vi "Process.vi"(8 "error in":errorcluster, 11 "DAQmx-AI":refnum<class "DAQmx-AI.lvclass">) -> (0 "error out":errorcluster, 3 "DAQmx-AI out":refnum<class "DAQmx-AI.lvclass">)   [LabVIEW 2016, in "DAQmx-AI.lvclass"]
doc: "---------------------------------------------------------------\nJKI State Machine Objects™\nhttp://jki.net/state-machine-objects/\nCopyright (C) 2005-2015, JKI <info@jki.net>\nALL RIGHTS RESERVEDJKI State Machine Objects (SMO) 1.0.0.5\nJKI - JKI\nCopyright (c) 2016, JKI"
uses:
  DAQmx-AI.lvclass
  C:/Program Files (x86)/National Instruments/LabVIEW 2016/vi.lib/JKI/JKI SMO/SMO/SMO.lvclass
  <vilib>/JKI/JKI SMO/SMO/Typedefs/Parent Call--Enum.ctl
  <vilib>/Platform/TimedLoop/XDataNode/timing_clust.ctl
  <vilib>/Platform/TimedLoop/XDataNode/nitl_modes.ctl
  <vilib>/Platform/TimedLoop/XDataNode/wakeup.ctl
  <vilib>/DAQmx/read.llb/DAQmx Read (Analog Wfm 1Chan NSamp).vi
  <vilib>/DAQmx/miscellaneous.llb/DAQmx Fill In Error Info.vi
  <vilib>/platform/TimedLoop/XDataNode/XDataNode.xnode
  <vilib>/JKI/JKI SMO/SMO/SMO.lvclass
  <vilib>/Platform/TimedLoop/XDataNode/XDNodeRunTimeDep.lvlib
panel:
  out "Chart":waveform(dbl)(graph)
  # "For instructions on how to use the JKI State Machine Objects, examples and video tutorials, visit:\nhttp://jki.net/state-machine-objects/\n\nJKI State Machine Objects™\nhttp://jki.net/state-machine-objects/\nCopyright (C) 2005-2015, JKI <info@jki.net>\nALL RIGHTS RESERVED"
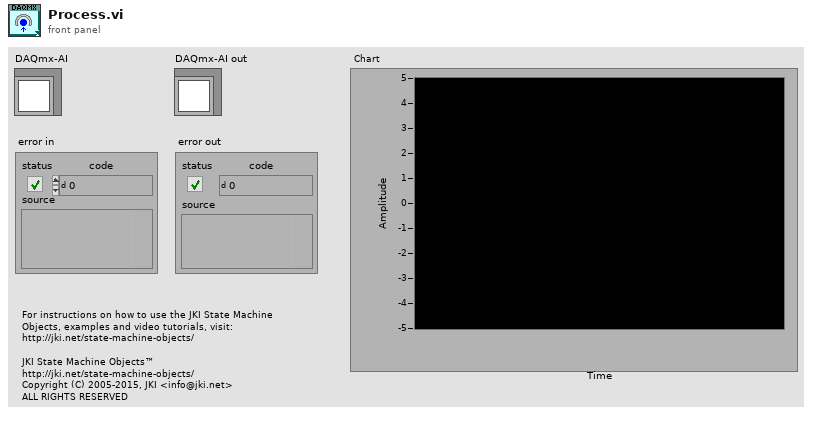
[diagram p1: front panel]
types:
  T1 = typedef "SMO.lvclass/Parent Call--Enum.ctl" = enum16{"Allows parent to run", "Does not request parent to run"}
  T2 = typedef "XDNodeRunTimeDep.lvlib/timing_clust.ctl" = cluster{"Expected End [f-1]":u64, "Actual End [f-1]":u64, "Finished Late? [f-1]":bool, "Expected End [i-1]":u64, "Actual End [i-1]":u64, "Finished Late? [i-1]":bool, "Expected Start [i]":u64, "Actual Start [i]":u64, "Expected Start [f]":u64, "Actual Start [f]":u64, "Source Name":string, "Structure Name":string, "Period":i64, "Deadline":i64, "Offset":i64, "Start":i64, "Priority":i32, "Timeout":i32, "Mode":T3, "Wakeup Reason":T4, "Error":errorcluster, "Source Type":string, "Secondary Source Type":string, "Global End Time":u64, "Global Start Time":u64, "Frame Duration":u64, "Iteration Duration":u64, "Assigned CPU":i32, "I/O Scan Engine Mode":u32}
  T3 = typedef "XDNodeRunTimeDep.lvlib/nitl_modes.ctl" = enum32{"No Change", "Process missed periods, maintain original phase", "Discard missed periods, maintain original phase", "Process missed periods, ignore original phase", "Discard missed periods, ignore original phase"}
  T4 = typedef "XDNodeRunTimeDep.lvlib/wakeup.ctl" = enum32{"Normal", "Aborted", "Asynchronous wakeup", "Timing source error", "Timed loop error", "Timeout"}
  T5 = typedef "SMO.lvclass/Protected Events.ctl" = cluster{"StopProcesses":refnum<user-event>, "AbortProcesses":refnum<user-event>, "Config Changed":refnum<user-event>, "Dependency":refnum<user-event>}
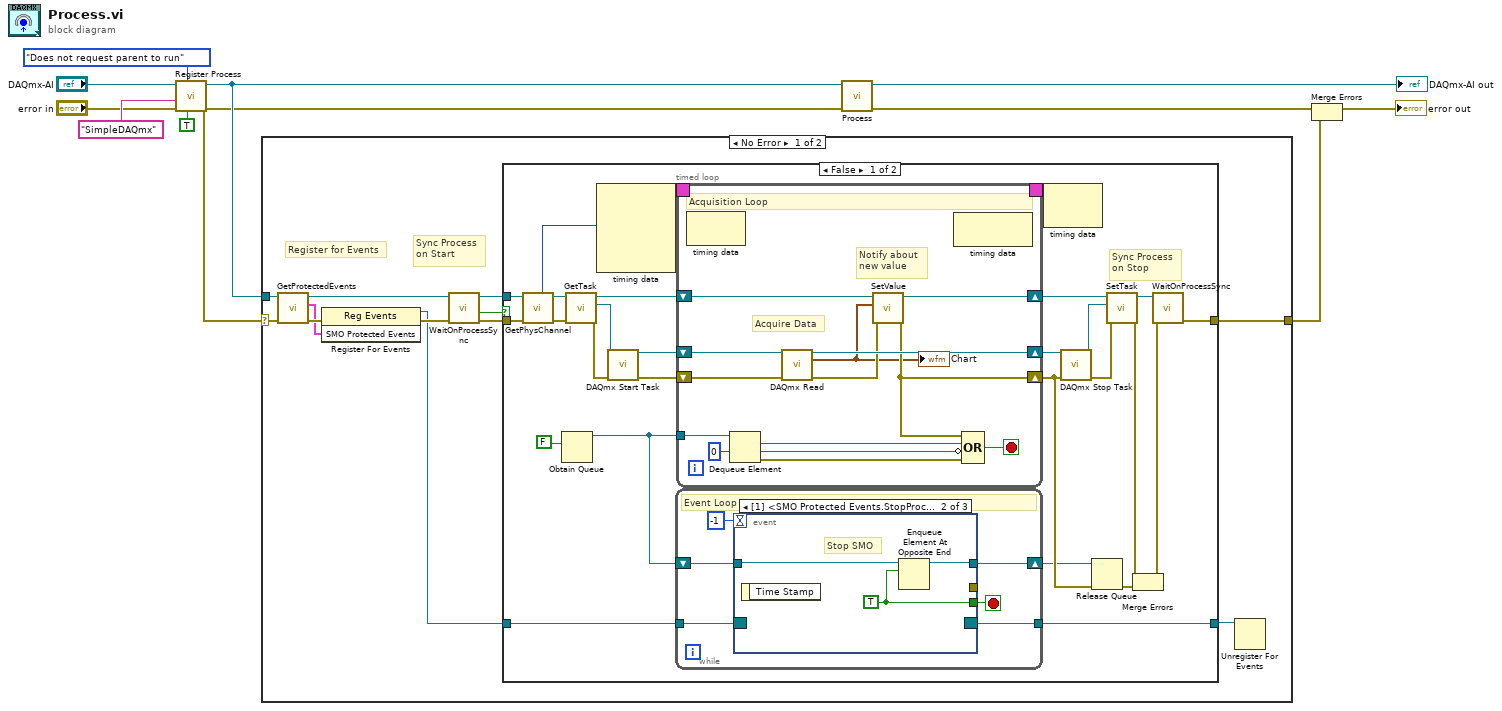
[diagram p0: block diagram]
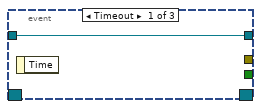
[diagram p2: hidden frame]
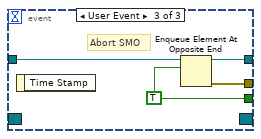
[diagram p3: hidden frame]
diagram:
  n1 = call <vilib>:"Register Process.vi"("Forces Self to Run (F)"=TRUE, "Parent Call"=Parent_Call--Enum."Does not request parent to run", "error in (no error)"="error in", "Process Name (optional)"="SimpleDAQmx", "SMO"="DAQmx-AI") -> ("error out"=w5:errorcluster, "SMO out"=w6:refnum<class "DAQmx-AI.lvclass">)  [unwired: 5 in]
  n2 = case shown="No Error" w5 {
    selector: w5 -> [w12 w87]
    tunnel: w6 -> [w13 _]
    tunnel: [w15 w87] -> w10
    frame No Error {
      # "Sync Process\non Start"
      # "Register for Events"
      n3 = call <vilib>:"GetProtectedEvents.vi"("error in (no error)"=w12, "SMO"=w13) -> ("error out"=w18:errorcluster, "SMO Protected Events"=w17:T5, "SMO out"=w19:refnum<class "DAQmx-AI.lvclass">)  [unwired: 7 in]
      n4 = register-events(error in=w18, w17) -> (reference out=w16:refnum<event-registration>, error out=w20:errorcluster)  [unwired: 1 in]
      n5 = call <vilib>:"WaitOnProcessSync.vi"("error in (no error)"=w20, "SMO"=w19) -> ("error out"=w22:errorcluster, "Don't run?"=w23:bool, "SMO out"=w21:refnum<class "DAQmx-AI.lvclass">)  [unwired: 7 in]
      n6 = case shown="False" w23 {
        tunnel: w22 -> [w45 w85]
        tunnel: w21 -> [w42 _]
        tunnel: w16 -> [w47 w86]
        tunnel: [w48 w85] -> w15
        tunnel: [w46 w86] -> w14
        frame False {
          # "Sync Process\non Stop"
          n7 = call "GetPhysChannel.vi"("error in (no error)"=w45, "DAQmx-AI"=w42) -> ("error out"=w31:errorcluster, "DAQmx-AI out"=w33:refnum<class "DAQmx-AI.lvclass">, "period (ms)"=w44:i64)  [unwired: 6 in, 1 out]
          n8 = Obtain Queue(element data type=FALSE) -> (queue out=w38:refnum<queue>)  [unwired: 4 in, 2 out]
          n9 = call "GetTask.vi"("error in (no error)"=w31, "DAQmx-AI"=w33) -> ("error out"=w29:errorcluster, "task"=w30:refnum<k21>, "DAQmx-AI out"=w32:refnum<class "DAQmx-AI.lvclass">)  [unwired: 7 in]
          n10 = node-c288(w44) -> (w50:T2)  [unwired: 3 in]
          n11 = call <vilib>:"DAQmx Start Task.vi"("task/channels in"=w30, "error in"=w29) -> ("task out"=w43:refnum<k21>, "error out"=w41:errorcluster)  [unwired: 12 in]
          n12 = while {
            tunnel: w47 -> [w55]
            tunnel: [w54] -> w46
            shift-right: [w51] -> w36
            shift-left: w38 -> [w52]
            stop <- w53 stop-if-true
            # "Event Loop"
            n13 = event shown="[1] <SMO Protected Events.StopProcesses>: User Event" {
              selector: w55 -> [_ _ _]
              dyn-events: [_ _ _] -> w54
              timeout: -1 -> [_ _ _]
              tunnel: [_ w59 w62] -> w53
              tunnel: w52 -> [w57 w60 w64]
              tunnel: [w57 w58 w63] -> w51
              tunnel: [_ _ w61] -> _
              event Timeout {
                n14 = event-data() -> ()  [unwired: 1 in, 1 out]
              }
              event User Event {
                w59 = TRUE
                # "Stop SMO"
                n15 = event-data() -> ()  [unwired: 1 in, 1 out]
                n16 = Enqueue Element At Opposite End(queue=w60, element=w59) -> (queue out=w58:refnum<queue>)  [unwired: 2 in, 2 out]
              }
              event User Event {
                w62 = TRUE
                # "Abort SMO"
                n17 = event-data() -> ()  [unwired: 1 in, 1 out]
                n18 = Enqueue Element At Opposite End(queue=w64, element=w62) -> (queue out=w63:refnum<queue>, error out=w61:errorcluster)  [unwired: 2 in, 1 out]
              }
            }
          }
          n19 = timed-loop {
            timing: w50 -> [_]
            timing-out: [_] -> w49
            tunnel: w38 -> [w70]
            shift-right: [w74] -> w40
            shift-left: w43 -> [w75]
            shift-right: [w76] -> w28
            shift-left: w32 -> [w77]
            shift-right: [w71] -> w37
            shift-left: w41 -> [w73]
            stop <- w78 stop-if-true
            # "Notify about\nnew value"
            # "Acquire Data"
            # "Acquisition Loop"
            n20 = node-c288() -> ()  [unwired: 1 in, 1 out]
            n21 = Dequeue Element(queue=w70, timeout in ms (-1)=0) -> (element=w68:bool, timed out?=w67:bool, error out=w66:errorcluster)  [unwired: 1 in, 1 out]
            n22 = call-poly <vilib>:"DAQmx Read.vi"("task/channels in"=w75, "error in"=w73) -> ("task out"=w74:refnum<k21>, "data"=w65:waveform(dbl), "error out"=w72:errorcluster)  [unwired: 11 in]
            "Chart" <- w65
            n23 = call "SetValue.vi"("error in (no error)"=w72, "Value"=w65, "DAQmx-AI"=w77) -> ("error out"=w71:errorcluster, "DAQmx-AI out"=w76:refnum<class "DAQmx-AI.lvclass">)  [unwired: 7 in]
            n24 = node-c288() -> ()  [unwired: 1 in, 1 out]
            n25 = Compound Arithmetic op=OR(w71, w68, invert w67, w66) -> (w78:bool)
          }
          n26 = node-c288(w49) -> ()  [unwired: 1 out]
          n27 = call <vilib>:"DAQmx Stop Task.vi"("task/channels in"=w40, "error in"=w37) -> ("task out"=w24:refnum<k21>, "error out"=w26:errorcluster)  [unwired: 12 in]
          n28 = Release Queue(queue=w36, error in (no error)=w37) -> (error out=w35:errorcluster)  [unwired: 1 in, 2 out]
          n29 = call "SetTask.vi"("error in (no error)"=w26, "task"=w24, "DAQmx-AI"=w28) -> ("error out"=w25:errorcluster, "DAQmx-AI out"=w27:refnum<class "DAQmx-AI.lvclass">)  [unwired: 7 in]
          n30 = Merge Errors(w25, w35) -> (w34:errorcluster)
          n31 = call <vilib>:"WaitOnProcessSync.vi"("error in (no error)"=w34, "SMO"=w27) -> ("error out"=w48:errorcluster)  [unwired: 7 in, 2 out]
        }
        frame True {
        }
      }
      n32 = Unregister For Events(event registration refnum=w14) -> ()  [unwired: 1 in, 1 out]
    }
    frame Error {
    }
  }
  n33 = call-parent "Process.vi"("error in"=w5, "SMO"=w6) -> ("error out"=w11:errorcluster, "SMO out"=→"DAQmx-AI out":refnum<class "DAQmx-AI.lvclass">)  [unwired: 8 in]
  n34 = Merge Errors(w11, w10) -> (→"error out":errorcluster)
